vi "Periodic Tasks.vi"(8 "error in":errorcluster) -> ()   [LabVIEW 2020]
doc: "This VI runs in parallel to other tasks. It can contain as many user-defined periodic loops as you need. These can carry out PID or other sorts of timed response."
uses:
  <vilib>/Rock Robotics/WPI/Ultrasonic/WPI_UltrasonicRangeUnits.ctl
  <vilib>/Rock Robotics/WPI/Utilities/WPI_GetSetVariantRefNum.vi
  <vilib>/Rock Robotics/WPI/Ultrasonic/WPI_SonarSRF04DigitalRefNum Registry Get.vi
  <vilib>/Rock Robotics/WPI/Ultrasonic/WPI_SonarSRF04DigitalGetRange.vi
  <vilib>/Rock Robotics/Network Tables/NT Write Number.vi
panel:
  out "left distance":dbl
  out "right distance":dbl
  out "front distance":dbl
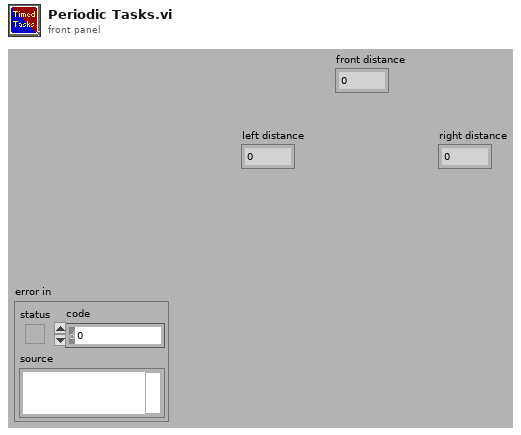
[diagram p1: front panel]
types:
  T1 = typedef "WPI_JoystickDevRef.ctl" = cluster{"Device":T2}
  T2 = typedef "WPI_JoystickDeviceEnum.ctl" = enum16{"USB 0", "USB 1", "USB 2", "USB 3", "USB 4", "USB 5"}
  T3 = typedef "WPI_RobotDriveDevRef.ctl" = cluster{"DevStatus":errorcluster, "Motors[]":T4[], "Square Inputs":bool, "Max Output":dbl}
  T4 = typedef "WPI_MotorControlDeviceRef.ctl" = cluster{"DeviceStatus":errorcluster, "Type":T5, "PWM":cluster{"PWM Channel":T6, "DeadBand":T7}, "CAN":cluster{"Device Number":u8, "SetOutput VI Ref":variant, "GetOutput VI Ref":variant, "Enable VI Ref":variant, "Disable VI Ref":variant, "Data":variant}, "Invert":bool, "DIO PWM":cluster{"PWM \"Enable\" Channel":T6, "DIOChannel":T8, "PWM Rate":dbl}}
  T5 = typedef "WPI_MotorControlType.ctl" = enum16{"PWM", "CAN", "DIO PWM"}
  T6 = typedef "FPGA_DIOPWMChannel.ctl" = enum8{"PWM 0", "PWM 1", "PWM 2", "PWM 3", "PWM 4", "PWM 5", "PWM 6", "PWM 7", "PWM 8", "PWM 9", "PWM MXP 0", "PWM MXP 1", "PWM MXP 2", "PWM MXP 3", "PWM MXP 4", "PWM MXP 5", "PWM MXP 6", "PWM MXP 7", "PWM MXP 8", "PWM MXP 9", "Invalid"}
  T7 = typedef "WPI_PWMDeadband.ctl" = cluster{"Name":string, "maxPositivePwm":i32, "minPositivePwm":i32, "centerPwm":i32, "maxNegativePwm":i32, "minNegativePwm":i32, "angularRange":u16}
  T8 = typedef "FPGA_DIOChannel.ctl" = enum8{"DIO 0", "DIO 1", "DIO 2", "DIO 3", "DIO 4", "DIO 5", "DIO 6", "DIO 7", "DIO 8", "DIO 9", "DIO MXP 0", "DIO MXP 1", "DIO MXP 2", "DIO MXP 3", "DIO MXP 4", "DIO MXP 5", "DIO MXP 6", "DIO MXP 7", "DIO MXP 8", "DIO MXP 9", "DIO MXP 10", "DIO MXP 11", "DIO MXP 12", "DIO MXP 13", "DIO MXP 14", "DIO MXP 15", "SPI Port CS1", "SPI Port CS2", "SPI Port CS3", "SPI Port MISO", "SPI Port MOSI", "Invalid"}
  T9 = typedef "WPI_UltrasonicDeviceRef.ctl" = cluster{"DevStatus":errorcluster, "Ping Channel":T8, "Echo Channel":T8, "CntIndex":T10}
  T10 = typedef "FPGA_CounterCtrSystemIndex.ctl" = enum8{"Ctr 0", "Ctr 1", "Ctr 2", "Ctr 3", "Ctr 4", "Ctr 5", "Ctr 6", "Ctr 7", "Invalid"}
  T11 = cluster{"JoystickDevRef":T1, "RobotDriveDevRef":T3}
  T12 = typedef "WPI_UltrasonicRangeUnits.ctl" = enum16{"inches", "mm"}
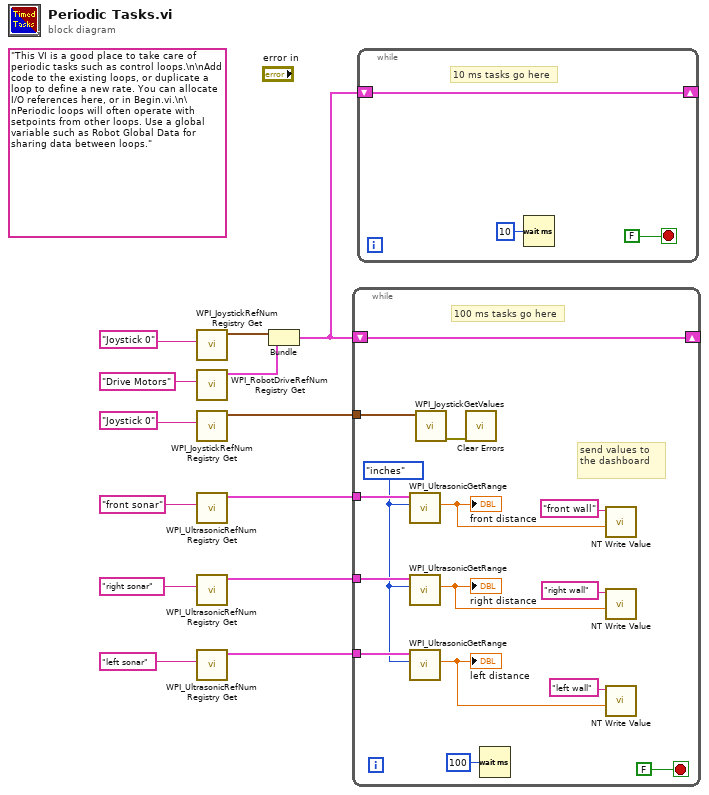
[diagram p0: block diagram]
diagram:
  (unwired) "This VI is a good place to take care of periodic tasks such as control loops.\n\nAdd code to the existing loops, or duplicate a loop to define a new rate. You can allocate I/O references here, or in Begin.vi.\n\nPeriodic loops will often operate with setpoints from other loops. Use a global variable such as Robot Global Data for sharing data between loops."
  n1 = call <vilib>:"WPI_JoystickRefNum Registry Get.vi"("refnum name"="Joystick 0") -> ("JoystickDevRef"=w11:T1)  [unwired: 1 in, 9 out]
  n2 = call <vilib>:"WPI_RobotDriveRefNum Registry Get.vi"("refnum name"="Drive Motors") -> ("RobotDriveDevRef"=w10:T3)  [unwired: 1 in, 9 out]
  n3 = call <vilib>:"WPI_JoystickRefNum Registry Get.vi"("refnum name"="Joystick 0") -> ("JoystickDevRef"=w7:T1)  [unwired: 1 in, 9 out]
  n4 = call-poly <vilib>:"WPI_UltrasonicRefNum Registry Get.vi"("refnum name"="front sonar") -> ("SonarSRF04DevRef"=w5:T9)  [unwired: 9 in, 1 out]
  n5 = call-poly <vilib>:"WPI_UltrasonicRefNum Registry Get.vi"("refnum name"="right sonar") -> ("SonarSRF04DevRef"=w4:T9)  [unwired: 9 in, 1 out]
  n6 = call-poly <vilib>:"WPI_UltrasonicRefNum Registry Get.vi"("refnum name"="left sonar") -> ("SonarSRF04DevRef"=w1:T9)  [unwired: 9 in, 1 out]
  n7 = Bundle("JoystickDevRef"=w11, "RobotDriveDevRef"=w10) -> (w9:T11)  [unwired: 1 out]
  n8 = while {
    shift-right: [w27] -> _
    shift-left: w9 -> [w27]
    tunnel: w7 -> [w26]
    tunnel: w5 -> [w25]
    tunnel: w4 -> [w24]
    tunnel: w1 -> [w23]
    stop <- FALSE stop-if-true
    w22 = WPI_UltrasonicRangeUnits."inches" ("Range Units")
    # "send values to the dashboard"
    # "100 ms tasks go here"
    n9 = call-poly <vilib>:"WPI_UltrasonicGetRange.vi"("ping time (s)"=w22, "UltrasonicDevRef"=w25) -> ("Distance"=w16:dbl)  [unwired: 7 in, 2 out]
    "front distance" <- w16
    n10 = call-poly <vilib>:"WPI_UltrasonicGetRange.vi"("ping time (s)"=w22, "UltrasonicDevRef"=w24) -> ("Distance"=w21:dbl)  [unwired: 7 in, 2 out]
    "right distance" <- w21
    n11 = call-poly <vilib>:"WPI_UltrasonicGetRange.vi"("ping time (s)"=w22, "UltrasonicDevRef"=w23) -> ("Distance"=w18:dbl)  [unwired: 7 in, 2 out]
    "left distance" <- w18
    n12 = call <vilib>:"WPI_JoystickGetValues.vi"("JoystickDevRef"=w26) -> ("error out"=w14:errorcluster)  [unwired: 6 in, 4 out]
    n13 = call <vilib>:"Clear Errors.vi"("error in (no error)"=w14) -> ()  [unwired: 5 in, 2 out]
    n14 = Wait (ms)(milliseconds to wait=u32 100) -> ()  [unwired: 1 out]
    n15 = call-poly <vilib>:"NT Write Value.vi"("Numeric"=w16, "Name"="front wall") -> ()  [unwired: 9 in, 1 out]
    n16 = call-poly <vilib>:"NT Write Value.vi"("Numeric"=w21, "Name"="right wall") -> ()  [unwired: 9 in, 1 out]
    n17 = call-poly <vilib>:"NT Write Value.vi"("Numeric"=w18, "Name"="left wall") -> ()  [unwired: 9 in, 1 out]
  }
  n18 = while {
    shift-right: [w29] -> _
    shift-left: w9 -> [w29]
    stop <- FALSE stop-if-true
    # "10 ms tasks go here"
    n19 = Wait (ms)(milliseconds to wait=u32 10) -> ()  [unwired: 1 out]
  }
